vi "valveStatus.vi"(8 "error in (no error)":errorcluster, 11 "VISA resource name":refnum<visa-resource-name>) -> (0 "error out":errorcluster, 1 "ValveClosed":bool, 2 "ValveOpen":bool, 3 "VISA resource name out":refnum<visa-resource-name>, 4 "Command status":string)   [LabVIEW 2012, in "ValveController.lvlib"]
uses:
  <instrlib>/ValveController/ValveController.lvlib
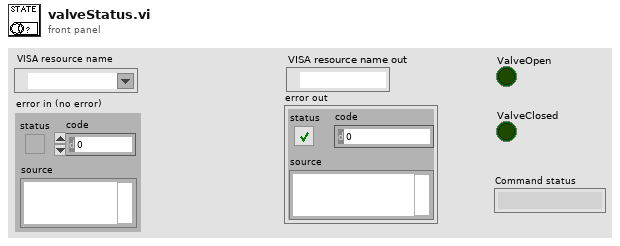
[diagram p1: front panel]
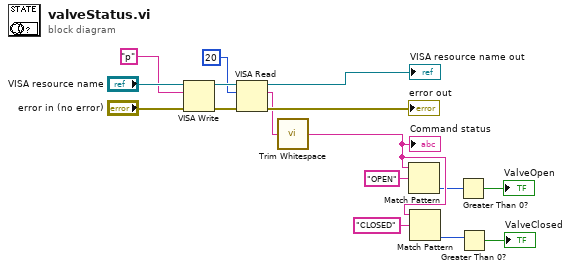
[diagram p0: block diagram]
diagram:
  n1 = VISA Write(VISA resource name="VISA resource name", write buffer="p", error in (no error)="error in (no error)") -> (VISA resource name out=w16:refnum<visa-resource-name>, error out=w15:errorcluster)  [unwired: 1 out]
  n2 = VISA Read(VISA resource name=w16, byte count=u32 20, error in (no error)=w15) -> (VISA resource name out=→"VISA resource name out":refnum<visa-resource-name>, read buffer=w8:string, error out=→"error out":errorcluster)  [unwired: 1 out]
  n3 = call <vilib>:"Trim Whitespace.vi"("string"=w8) -> ("trimmed string"=w5:string)  [unwired: 1 in]
  "Command status" <- w5
  n4 = Match Pattern(string=w5, regular expression="OPEN") -> (offset past match=w4:i32)  [unwired: 1 in, 3 out]
  n5 = Match Pattern(string=w5, regular expression="CLOSED") -> (offset past match=w1:i32)  [unwired: 1 in, 3 out]
  n6 = Greater Than 0?(x=w4) -> (x > 0?=→"ValveOpen":bool)
  n7 = Greater Than 0?(x=w1) -> (x > 0?=→"ValveClosed":bool)
